vi "GetThresholdChannels.vi"(11 "Sensor Info":string[][](array[string])) -> (0 "ThresholdValue":dbl[](array[numeric]), 1 "IsMinThreshold":bool[](array[boolean]), 2 "RPM Engage":dbl[](array[numeric]), 3 "ThresholdChannels":string[](array[string]))   [LabVIEW 2018, in "Controller (Host).lvlib"]
uses:
  Controller (Host).lvlib
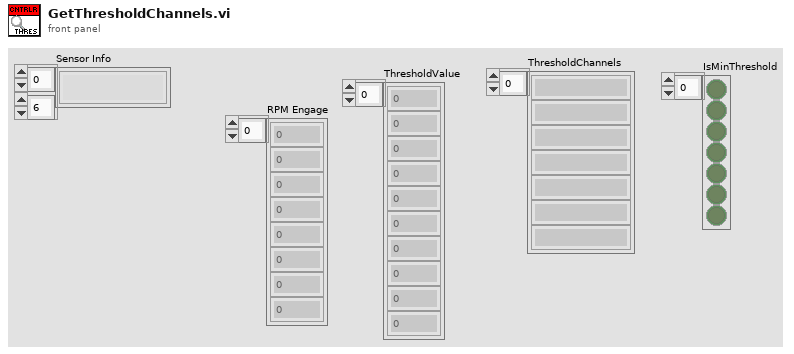
[diagram p1: front panel]
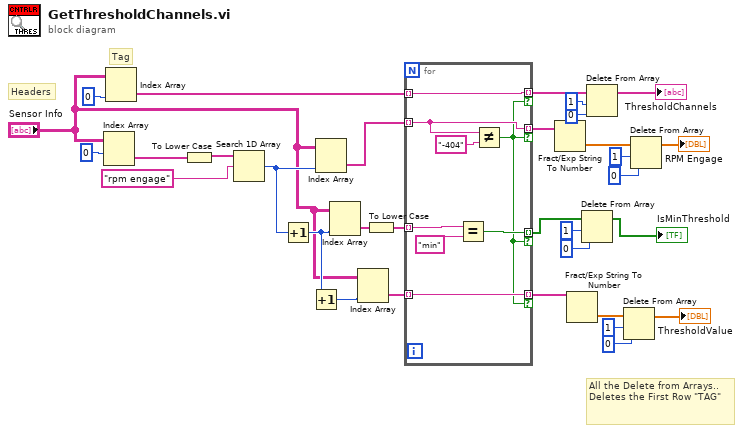
[diagram p0: block diagram]
diagram:
  # "All the Delete from Arrays..\nDeletes the First Row \"TAG\""
  # "Tag"
  # "Headers"
  n1 = Index Array(array="Sensor Info", index (row)=0) -> (element=w26:string[])  [unwired: 1 in]
  n2 = Index Array(array="Sensor Info", index (col)=0 ("disabled index (col)")) -> (element=w31:string[])  [unwired: 1 in]
  n3 = To Lower Case(string=w26) -> (all lower case string=w28:string[])
  n4 = Search 1D Array(1D array=w28, element="rpm engage") -> (index of element=w29:i32)  [unwired: 1 in]
  n5 = Increment(x=w29) -> (x+1=w18:i32)
  n6 = Increment(x=w18) -> (x+1=w19:i32)
  n7 = Index Array(array="Sensor Info", index (col)=w29) -> (element=w23:string[])  [unwired: 1 in]
  n8 = Index Array(array="Sensor Info", index (col)=w18) -> (element=w21:string[])  [unwired: 1 in]
  n9 = Index Array(array="Sensor Info", index (col)=w19) -> (element=w16:string[])  [unwired: 1 in]
  n10 = To Lower Case(string=w21) -> (all lower case string=w20:string[])
  n11 = for {
    tunnel: w23 -> [w38] mode=indexing
    tunnel: w31 -> [w39] mode=indexing
    tunnel: [w39] -> w32 mode=indexing if=w33
    tunnel: [w38] -> w22 mode=indexing if=w33
    tunnel: w20 -> [w37] mode=indexing
    tunnel: [w36] -> w8 mode=indexing if=w33
    tunnel: w16 -> [w34] mode=indexing
    tunnel: [w34] -> w15 mode=indexing if=w33
    n12 = Equal?(x=w37, y="min") -> (x = y?=w36:bool)
    n13 = Not Equal?(x=w38, y="-404" ("t")) -> (x != y?=w33:bool)
  }
  n14 = Fract/Exp String To Number(string=w22) -> (number=w24:dbl[])  [unwired: 3 in, 1 out]
  n15 = Fract/Exp String To Number(string=w15) -> (number=w14:dbl[])  [unwired: 3 in, 1 out]
  n16 = Delete From Array(array=w8, length=1, index=0) -> (array with subset deleted=→"IsMinThreshold":bool[])  [unwired: 1 out]
  n17 = Delete From Array(array=w32, length=1, index=0) -> (array with subset deleted=→"ThresholdChannels":string[])  [unwired: 1 out]
  n18 = Delete From Array(array=w14, length=1, index=0) -> (array with subset deleted=→"ThresholdValue":dbl[])  [unwired: 1 out]
  n19 = Delete From Array(array=w24, length=1, index=0) -> (array with subset deleted=→"RPM Engage":dbl[])  [unwired: 1 out]
